vi "Convert FLI Parameters v2 to v3.vi"(1 "FLI Parameters v2":T1) -> (0 "FLI Parameters v3":T2)   [LabVIEW 2021, in "Phasor.lvlib"]
uses:
  Phasor Fluorescence Lifetime Parameters v3.ctl
  Phasor Fluorescence Lifetime Parameters v2.ctl
  Phasor.lvlib
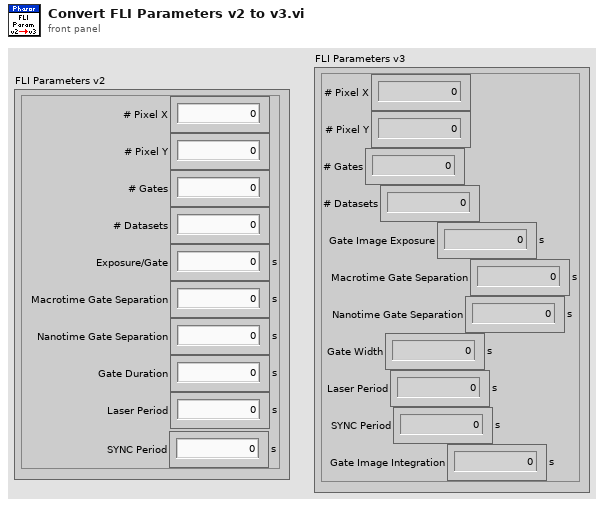
[diagram p1: front panel]
types:
  T1 = typedef "Phasor.lvlib/Phasor Fluorescence Lifetime Parameters v2.ctl" = cluster{"# Pixel X":i32, "# Pixel Y":i32, "# Gates":i32, "# Datasets":i32, "Exposure/Gate":dbl[unit], "Macrotime Gate Separation":dbl[unit], "Nanotime Gate Separation":dbl[unit], "Gate Duration":dbl[unit], "Laser Period":dbl[unit], "SYNC Period":dbl[unit]}
  T2 = typedef "Phasor.lvlib/Phasor Fluorescence Lifetime Parameters v3.ctl" = cluster{"# Pixel X":i32, "# Pixel Y":i32, "# Gates":i32, "# Datasets":i32, "Gate Image Exposure":dbl[unit], "Macrotime Gate Separation":dbl[unit], "Nanotime Gate Separation":dbl[unit], "Gate Width":dbl[unit], "Laser Period":dbl[unit], "SYNC Period":dbl[unit], "Gate Image Integration":dbl[unit]}
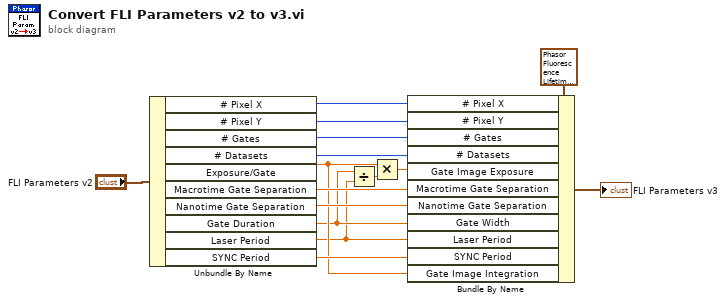
[diagram p0: block diagram]
diagram:
  n1 = Unbundle By Name("FLI Parameters v2") -> ("# Pixel X"=w14:i32, "# Pixel Y"=w12:i32, "# Gates"=w11:i32, "# Datasets"=w10:i32, "Exposure/Gate"=w5:dbl[unit], "Macrotime Gate Separation"=w9:dbl[unit], "Nanotime Gate Separation"=w8:dbl[unit], "Gate Duration"=w4:dbl[unit], "Laser Period"=w3:dbl[unit], "SYNC Period"=w7:dbl[unit])
  n2 = Divide(x=w4, y=w3) -> (x/y=w2:dbl)
  n3 = Multiply(x=w5, y=w2) -> (x*y=w1:dbl[unit])
  n4 = Bundle By Name(cluster=T2 {"# Pixel X"=0, "# Pixel Y"=0, "# Gates"=0, "# Datasets"=0, "Gate Image Exposure"=0.0, "Macrotime Gate Separation"=0.0, "Nanotime Gate Separation"=0.0, "Gate Width"=0.0, "Laser Period"=0.0, "SYNC Period"=0.0, "Gate Image Integration"=0.0} ("FLI Parameters v2"), "# Pixel X"=w14, "# Pixel Y"=w12, "# Gates"=w11, "# Datasets"=w10, "Gate Image Exposure"=w1, "Macrotime Gate Separation"=w9, "Nanotime Gate Separation"=w8, "Gate Width"=w4, "Laser Period"=w3, "SYNC Period"=w7, "Gate Image Integration"=w5) -> (→"FLI Parameters v3":T2)
